vi "G# - Property Example LV2009.vi"() -> ()   [LabVIEW 2020]
doc: "Property\nThis example shows how properties are used in LV2009."
uses:
  MyPropertyClass_LV2009_class/MyPropertyClass_LV2009.lvclass
  vi.lib/addons/_AddQ/G#Object/G#Object.lvclass
panel:
  out "Name out":string
  in  "error in (no error)":errorcluster
  out "error out":errorcluster
  in  "Name":string="AddQ"
  # "Property\nThis example shows how properties are used in LV2009."
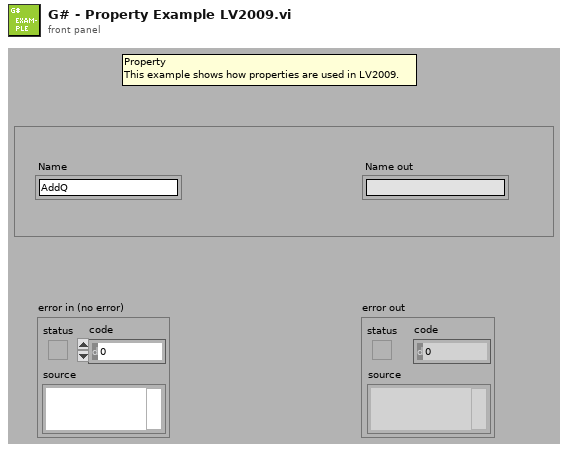
[diagram p1: front panel]
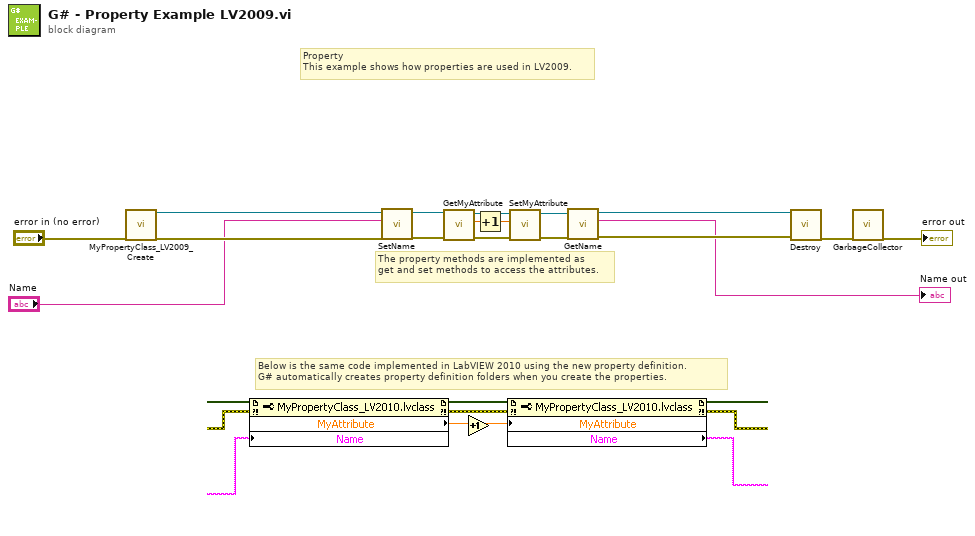
[diagram p0: block diagram]
diagram:
  # "Below is the same code implemented in LabVIEW 2010 using the new property definition.\nG# automatically creates property definition folders when you create the properties."
  # "The property methods are implemented as\nget and set methods to access the attributes."
  # "Property\nThis example shows how properties are used in LV2009."
  n1 = call "MyPropertyClass_LV2009_Create.vi"("error in (no error)"="error in (no error)") -> ("reference out"=w17:refnum<class "MyPropertyClass_LV2009.lvclass">, "error out"=w16:errorcluster)  [unwired: 17 in]
  n2 = call-dynamic "SetName.vi"("error in (no error)"=w16, "Name"="Name", "reference in"=w17) -> ("error out"=w8:errorcluster, "reference out"=w7:refnum<class "MyPropertyClass_LV2009.lvclass">)  [unwired: 7 in]
  n3 = call-dynamic "GetMyAttribute.vi"("error in (no error)"=w8, "reference in"=w7) -> ("error out"=w6:errorcluster, "MyAttribute"=w4:dbl, "reference out"=w5:refnum<class "MyPropertyClass_LV2009.lvclass">)  [unwired: 7 in]
  n4 = Increment(x=w4) -> (x+1=w1:dbl)
  n5 = call-dynamic "SetMyAttribute.vi"("error in (no error)"=w6, "MyAttribute"=w1, "reference in"=w5) -> ("error out"=w3:errorcluster, "reference out"=w2:refnum<class "MyPropertyClass_LV2009.lvclass">)  [unwired: 7 in]
  n6 = call-dynamic "GetName.vi"("error in (no error)"=w3, "reference in"=w2) -> ("error out"=w13:errorcluster, "Name"=→"Name out":string, "reference out"=w14:refnum<class "MyPropertyClass_LV2009.lvclass">)  [unwired: 7 in]
  n7 = call-dynamic "Destroy.vi"("reference in"=w14, "error in (no error)"=w13) -> ("error out"=w10:errorcluster)  [unwired: 16 in, 1 out]
  n8 = call "GarbageCollector.vi"("error in (no error)"=w10) -> ("error out"=→"error out":errorcluster)  [unwired: 16 in, 2 out]
